vi "Set Bricks Positions.vi"(8 "error in (no error)":errorcluster, 10 "Brick Wall":T1[](array[typedef]), 11 "object in":refnum<class "Wall.lvclass">) -> (0 "error out":errorcluster, 3 "object out":refnum<class "Wall.lvclass">)   [LabVIEW 2017, in "Wall.lvclass"]
uses:
  Wall.lvclass
  Controls/Coordinates.ctl
  Wall.lvclass/Wall.ctl
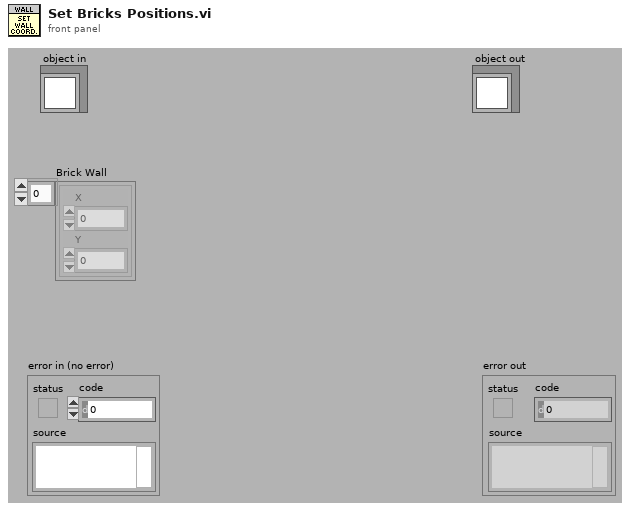
[diagram p1: front panel]
types:
  T1 = typedef "Coordinates.ctl" = cluster{"X":i32, "Y":i32}
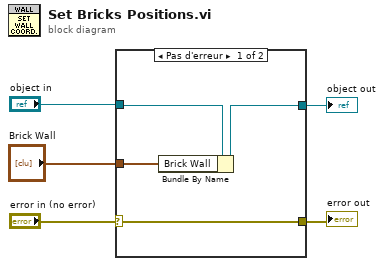
[diagram p0: block diagram]
diagram:
  n1 = case shown="Pas d'erreur" "error in (no error)" {
    selector: "error in (no error)" -> [w9 w11]
    tunnel: [w9 w11] -> w4
    tunnel: [w7 w10] -> w2
    tunnel: "object in" -> [w8 w10]
    tunnel: "Brick Wall" -> [w6 _]
    frame No Error {
      n2 = Bundle By Name(cluster=w8, "Brick Wall"=w6) -> (w7:refnum<class "Wall.lvclass">)
    }
    frame Error {
    }
  }
  "error out" <- w4
  "object out" <- w2
